vi "Format Waveform and Send.vi"(8 "error in (no error)":errorcluster, 10 "Waveform Array":sgl[][](array[numeric]), 11 "DAQ Actor in":refnum<class "DAQ Actor.lvclass">) -> (0 "error out":errorcluster, 3 "DAQ Actor out":refnum<class "DAQ Actor.lvclass">)   [LabVIEW 2018, in "Data Acquisition.lvlib" / "DAQ Actor.lvclass"]
uses:
  DAQ Actor.lvclass
  DAQ Actor.lvclass/DAQ Actor.ctl
  TCP Server/TCP Writer Messages/Write Data to Stream Msg/Write Data to Conn Msg.lvclass/Write Data to Conn Msg.ctl
  <vilib>/ActorFramework/Message Enqueuer/Message Enqueuer.lvclass/Message Enqueuer.ctl
  <vilib>/ActorFramework/Message Enqueuer/Enqueue.vi
  TCP Server/TCP Writer Messages/Write Data to Stream Msg/Write Data to Conn Msg.lvclass
  C:/Program Files (x86)/National Instruments/LabVIEW 2018/vi.lib/ActorFramework/Message/Message.lvclass
  <vilib>/ActorFramework/Message Priority Queue/Priority Enqueue.vi
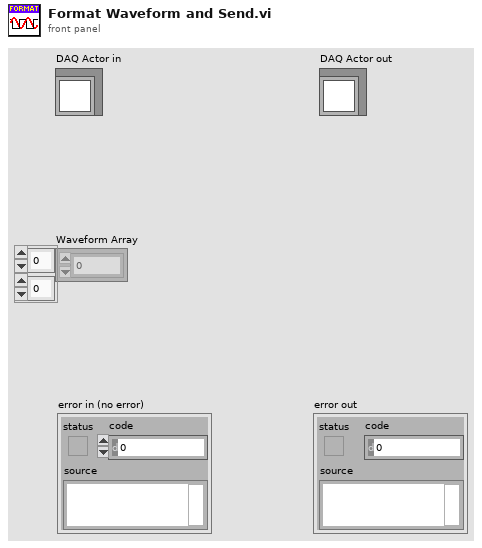
[diagram p1: front panel]
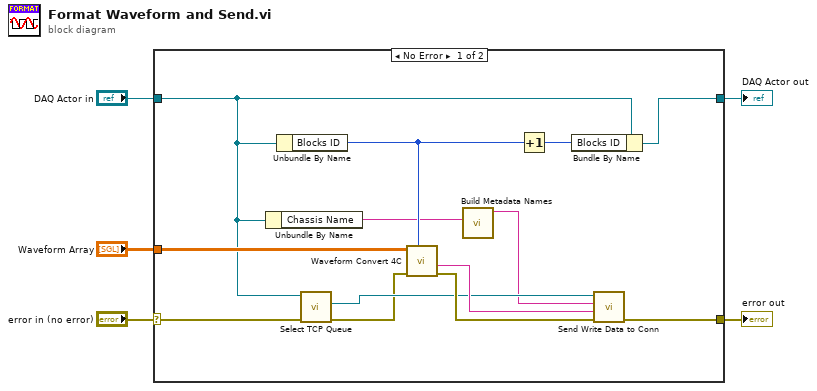
[diagram p0: block diagram]
diagram:
  n1 = case shown="No Error" "error in (no error)" {
    selector: "error in (no error)" -> [w14 w20]
    tunnel: [w18 w20] -> w5
    tunnel: "Waveform Array" -> [w17 _]
    tunnel: "DAQ Actor in" -> [w15 w19]
    tunnel: [w16 w19] -> w1
    frame No Error {
      n2 = Unbundle By Name(w15) -> ("Chassis Name"=w7:string)
      n3 = Unbundle By Name(w15) -> ("Blocks ID"=w10:u32)
      n4 = call "Select TCP Queue.vi"("error in (no error)"=w14, "DAQ Actor in"=w15) -> ("error out"=w8:errorcluster, "TCP Queue"=w9:refnum<class "Message Enqueuer.lvclass">)  [unwired: 7 in, 1 out]
      n5 = call "Waveform Convert 4C.vi"("BlockID"=w10, "error in"=w8, "Waveform Array"=w17) -> ("error out"=w12:errorcluster, "ModWfms"=w13:string)  [unwired: 7 in]
      n6 = call "Build Metadata Names.vi"("Chassis Name"=w7) -> ("Wfm"=w6:string)  [unwired: 6 in, 4 out]
      n7 = Increment(x=w10) -> (x+1=w11:u32)
      n8 = Bundle By Name(cluster=w15, "Blocks ID"=w11) -> (w16:refnum<class "DAQ Actor.lvclass">)
      n9 = call "Send Write Data to Conn.vi"("error in (no error)"=w12, "Data"=w13, "MetaData"=w6, "Message Enqueuer"=w9) -> ("error out"=w18:errorcluster)  [unwired: 6 in, 1 out]
    }
    frame Error {
    }
  }
  "error out" <- w5
  "DAQ Actor out" <- w1
